vi "fields delete field.vi"(4 "User":T1, 8 "error in (no error)":errorcluster, 9 "Field_ID (\"\")":string, 11 "Connection Refnum":T2) -> (0 "error out":errorcluster, 3 "Connection Refnum":T2)   [LabVIEW 2011]
uses:
  SI.LIB/ODBC/SQL Controls/Connection Refnum.ctl
  server/database/Users/User Record.ctl
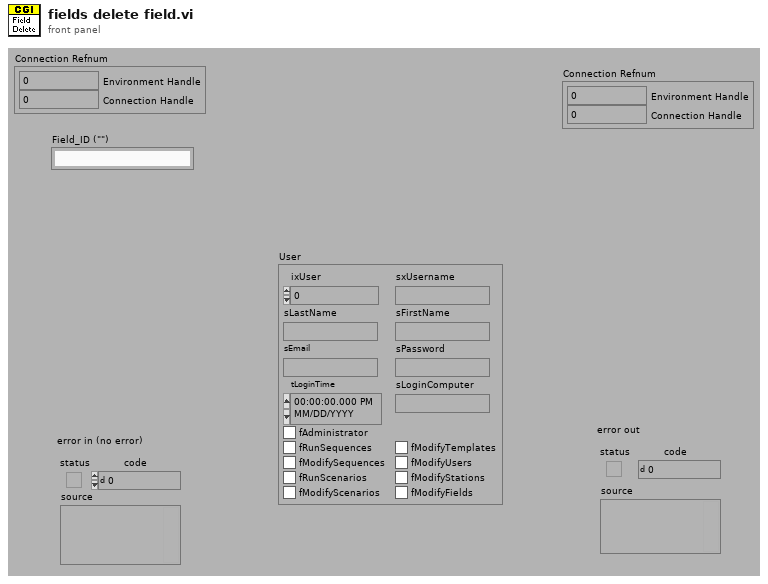
[diagram p1: front panel]
types:
  T1 = typedef "User Record.ctl" = cluster{"ixUser":i32, "sxUsername":string, "sLastName":string, "sFirstName":string, "sEmail":string, "sPassword":string, "tLoginTime":timestamp, "sLoginComputer":string, "fAdministrator":bool, "fRunSequences":bool, "fModifySequences":bool, "fRunScenarios":bool, "fModifyScenarios":bool, "fModifyTemplates":bool, "fModifyUsers":bool, "fModifyStations":bool, "fModifyFields":bool}
  T2 = typedef "Connection Refnum.ctl" = cluster{"Environment Handle":i32, "Connection Handle":i32}
  T3 = typedef "Field Record.ctl" = cluster{"ixField":i32, "iSequenceOrder":i32, "sxFieldId":string, "sxSequenceId":string, "sDisplayName":string, "sValue":string, "sUnits":string, "nDataType":T4, "nNextItem":T5, "fSystem":bool, "fSystemValue":bool, "fRequired":bool, "fSetAtTest":bool, "fTestField":bool, "fDeleted":bool, "fIndexed":bool, "fFreeList":bool}
  T4 = typedef "Field DataTypes.ctl" = enum32{"text", "numeric", "list", "timestamp", "boolean"}
  T5 = typedef "Field NextItem.ctl" = enum32{"Reset", "Retain", "Auto-Increment"}
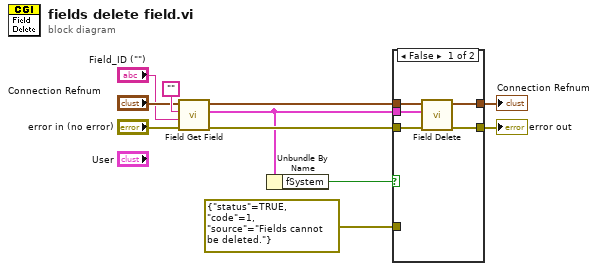
[diagram p0: block diagram]
diagram:
  n1 = call "Field Get Field.vi"("error in (no error)"="error in (no error)", "sFieldId or sDisplayName (\"\")"="Field_ID (\"\")", "sxSequenceId (\"\")"="", "Connection Refnum"="Connection Refnum") -> ("error out"=w11:errorcluster, "Field"=w3:T3, "Connection Refnum"=w10:T2)  [unwired: 1 in, 4 out]
  n2 = Unbundle By Name(w3) -> ("fSystem"=w1:bool)
  n3 = case shown="False" w1 {
    tunnel: w11 -> [w16 _]
    tunnel: w10 -> [w15 w18]
    tunnel: [w14 w18] -> w5
    tunnel: [w13 w17] -> w4
    tunnel: w3 -> [w12 _]
    tunnel: errorcluster {"status"=TRUE, "code"=1, "source"="Fields cannot be deleted."} ("error out") -> [_ w17]
    frame False {
      n4 = call "Field Delete.vi"("error in (no error)"=w16, "Field"=w12, "Connection Refnum"=w15) -> ("error out"=w13:errorcluster, "Connection Refnum"=w14:T2)  [unwired: 7 out]
    }
    frame True {
    }
  }
  "error out" <- w4
  "Connection Refnum" <- w5
